vi "intersecAreaQuad.vi"(8 "error in (no error)":errorcluster, 9 "Ball/Enemy\nPosition":dbl[](array[numeric]), 10 "Game":refnum<class "Game.lvclass">, 11 "Utilities in":refnum<class "Utilities.lvclass">) -> (0 "error out":errorcluster, 1 "Game":refnum<class "Game.lvclass">, 2 "Pos de Interseção":dbl[](array[numeric]) format="%#_13g", 3 "Utilities out":refnum<class "Utilities.lvclass">)   [LabVIEW 2023, in "Utilities.lvclass"]
uses:
  Utilities.lvclass
  Game_class/Game.lvclass
  Game_class/Game.lvclass/Game.ctl
  Game_class/Read FieldRef.vi
  Field_class/Field.lvclass
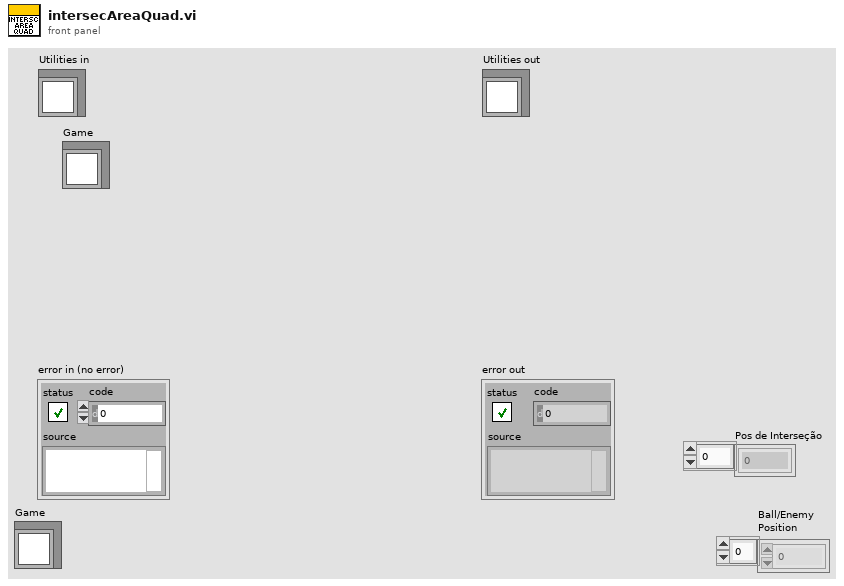
[diagram p1: front panel]
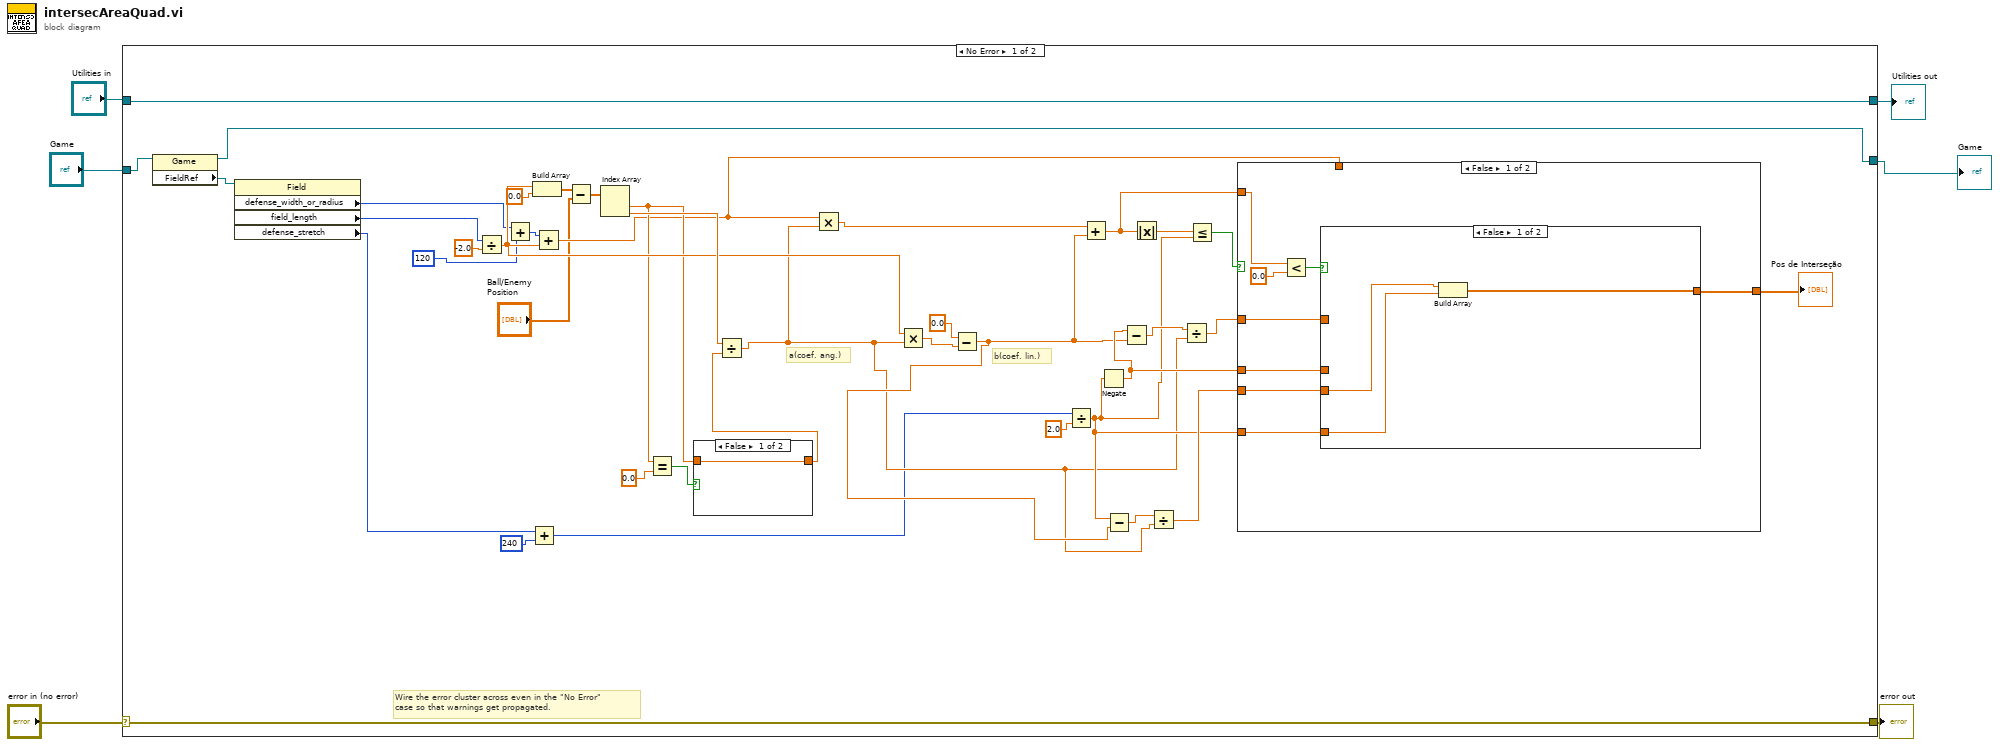
[diagram p0: block diagram]
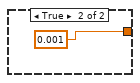
[diagram p2: hidden frame]
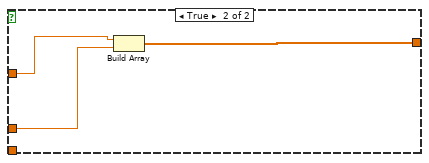
[diagram p3: hidden frame]
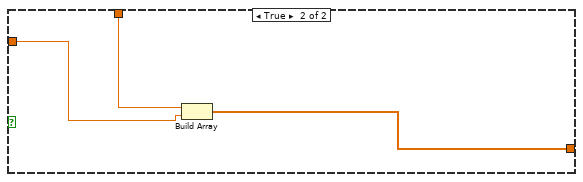
[diagram p4: hidden frame]
diagram:
  n1 = case shown="No Error" "error in (no error)" {
    selector: "error in (no error)" -> [w45 w67]
    tunnel: [w45 w67] -> w5
    tunnel: [w46 w66] -> w3
    tunnel: "Utilities in" -> [w46 w66]
    tunnel: "Game" -> [w13 _]
    tunnel: [w7 _] -> w1
    frame No Error {
      # "b(coef. lin.)"
      # "a(coef. ang.)"
      # "Wire the error cluster across even in the \"No Error\"\ncase so that warnings get propagated."
      n2 = property class="Game"(reference=w13) -> (reference out=w7:refnum<class "Game.lvclass">, "FieldRef"=w12:refnum<class "Field.lvclass">)  [unwired: 1 in, 1 out]
      n3 = property class="Field"(reference=w12) -> ("defense_width_or_radius"=w11:i32, "field_length"=w10:i32, "defense_stretch"=w9:i32)  [unwired: 1 in, 2 out]
      n4 = Divide(x=w10, y=-2.0) -> (x/y=w37:dbl)
      n5 = Add(x=w11, y=u32 120) -> (x+y=w16:u32)
      n6 = Add(x=w9, y=u32 240) -> (x+y=w15:u32)
      n7 = Build Array(w37, 0.0 ("element")) -> (w42:dbl[])
      n8 = Add(x=w16, y=w37) -> (x+y=w18:dbl)
      n9 = Subtract(x=w42, y="Ball/Enemy\nPosition") -> (x-y=w41:dbl[])
      n10 = Index Array(array=w41) -> (element #1=w22:dbl, element #2=w40:dbl)  [unwired: 2 in]
      n11 = Equal?(x=w22, y=0.0) -> (x = y?=w23:bool)
      n12 = case shown="False" w23 {
        tunnel: w22 -> [w47 _]
        tunnel: [w47 0.001] -> w21
        frame False {
        }
        frame True {
        }
      }
      n13 = Divide(x=w40, y=w21) -> (x/y=w25:dbl)
      n14 = Multiply(x=w18, y=w25) -> (x*y=w36:dbl)
      n15 = Multiply(x=w37, y=w25) -> (x*y=w39:dbl)
      n16 = Subtract(x=0.0, y=w39) -> (x-y=w29:dbl)
      n17 = Divide(x=w15, y=2.0) -> (x/y=w26:dbl)
      n18 = Add(x=w36, y=w29) -> (x+y=w17:dbl)
      n19 = Negate(x=w26) -> (-x=w30:dbl)
      n20 = Subtract(x=w26, y=w29) -> (x-y=w28:dbl)
      n21 = Subtract(x=w30, y=w29) -> (x-y=w32:dbl)
      n22 = Absolute Value(x=w17) -> (abs(x)=w35:dbl)
      n23 = Divide(x=w28, y=w25) -> (x/y=w27:dbl)
      n24 = Divide(x=w32, y=w25) -> (x/y=w31:dbl)
      n25 = Less Or Equal?(x=w35, y=w26) -> (x <= y?=w33:bool)
      n26 = case shown="False" w33 {
        tunnel: w17 -> [w56 w63]
        tunnel: w18 -> [_ w64]
        tunnel: [w51 w65] -> w14
        tunnel: w31 -> [w53 _]
        tunnel: w30 -> [w52 _]
        tunnel: w27 -> [w50 _]
        tunnel: w26 -> [w49 _]
        frame False {
          n27 = Less?(x=w56, y=0.0) -> (x < y?=w54:bool)
          n28 = case shown="False" w54 {
            tunnel: w53 -> [_ w61]
            tunnel: w52 -> [_ w60]
            tunnel: [w59 w62] -> w51
            tunnel: w50 -> [w58 _]
            tunnel: w49 -> [w57 _]
            frame False {
              n29 = Build Array(w58, w57) -> (w59:dbl[])
            }
            frame True {
              n30 = Build Array(w61, w60) -> (w62:dbl[])
            }
          }
        }
        frame True {
          n31 = Build Array(w64, w63) -> (w65:dbl[])
        }
      }
      "Pos de Interseção" <- w14
    }
    frame Error {
    }
  }
  "error out" <- w5
  "Utilities out" <- w3
  "Game" <- w1
